vi "PLC_Main_Screen_communication.vi"() -> ()   [LabVIEW 2017]
doc: "Andon System cards scanning and ouput ON/OFF through MQTT protocol. Update data in SQL data base for reporting."
uses:
  Control/Processing_enum.ctl
  Control/Main_Data.ctl
  Control/Andon_demo State.ctl
  <vilib>/addons/database/Connection.llb/Conn ObjectReference.ctl
  <vilib>/NI/Modbus Library/API/master/Modbus Master.lvclass
  Control/Oven_State.ctl
  37ed035b-2b4a-44e1-bf61-a1f42ff74949.vi
  <vilib>/addons/database/Connection.llb/DB Tools Open Connec (Path).vi
  <vilib>/NI/Modbus Library/API/Wrapper/Create TCP Master.vi
  <vilib>/ethernetip/ethernetip.llb/EthernetIP SLC500 Read Bit.vi
  <vilib>/ethernetip/ethernetip.llb/EthernetIP SLC500 Write Bit.vi
  <vilib>/addons/database/NI_Database_API.lvlib
  <vilib>/ethernetip/ethernetip.lvlib
  <vilib>/NI/Modbus Library/API/Wrapper/API Main.lvlib
panel:
  in  "stop":bool
  out "Stop from Main":bool
  out "Change Element":T1(array[cluster])
  out "MACHINE NAME":string[](array[string])
  out "IP Address":string[](array[string])
  in  "Tab Control":enum32{"Oven", "press"}(tab)
  out "Oven Values":u16[][](array[numeric])
  out "Oven live Sql Error":errorcluster
  out "Oven Station ID":string[][](array[string])
  out "Oven LOG SQL Error":errorcluster
  out "LOG Elapsed Time":dbl caption="Elapsed Time (s)"
  out "output cluster":T2
  out "Press Statio ID":string[][](array[string])
  out "Cluster":T3
  out "STATE":T4=enum."PLC_stat"
  out "Shift":i32
  out "CID":string
  out "error out":errorcluster
  out "Deq Element":T5[](array[typedef])
  out "PLC Data":T5[](array[typedef])
  out "Input":bool[](array[boolean])
  # "SERVER for PRESS and OVEN"
  # "1.INPUTS\n2.OUTPUTS\n3.Product code running on system.\n4.Alarms"
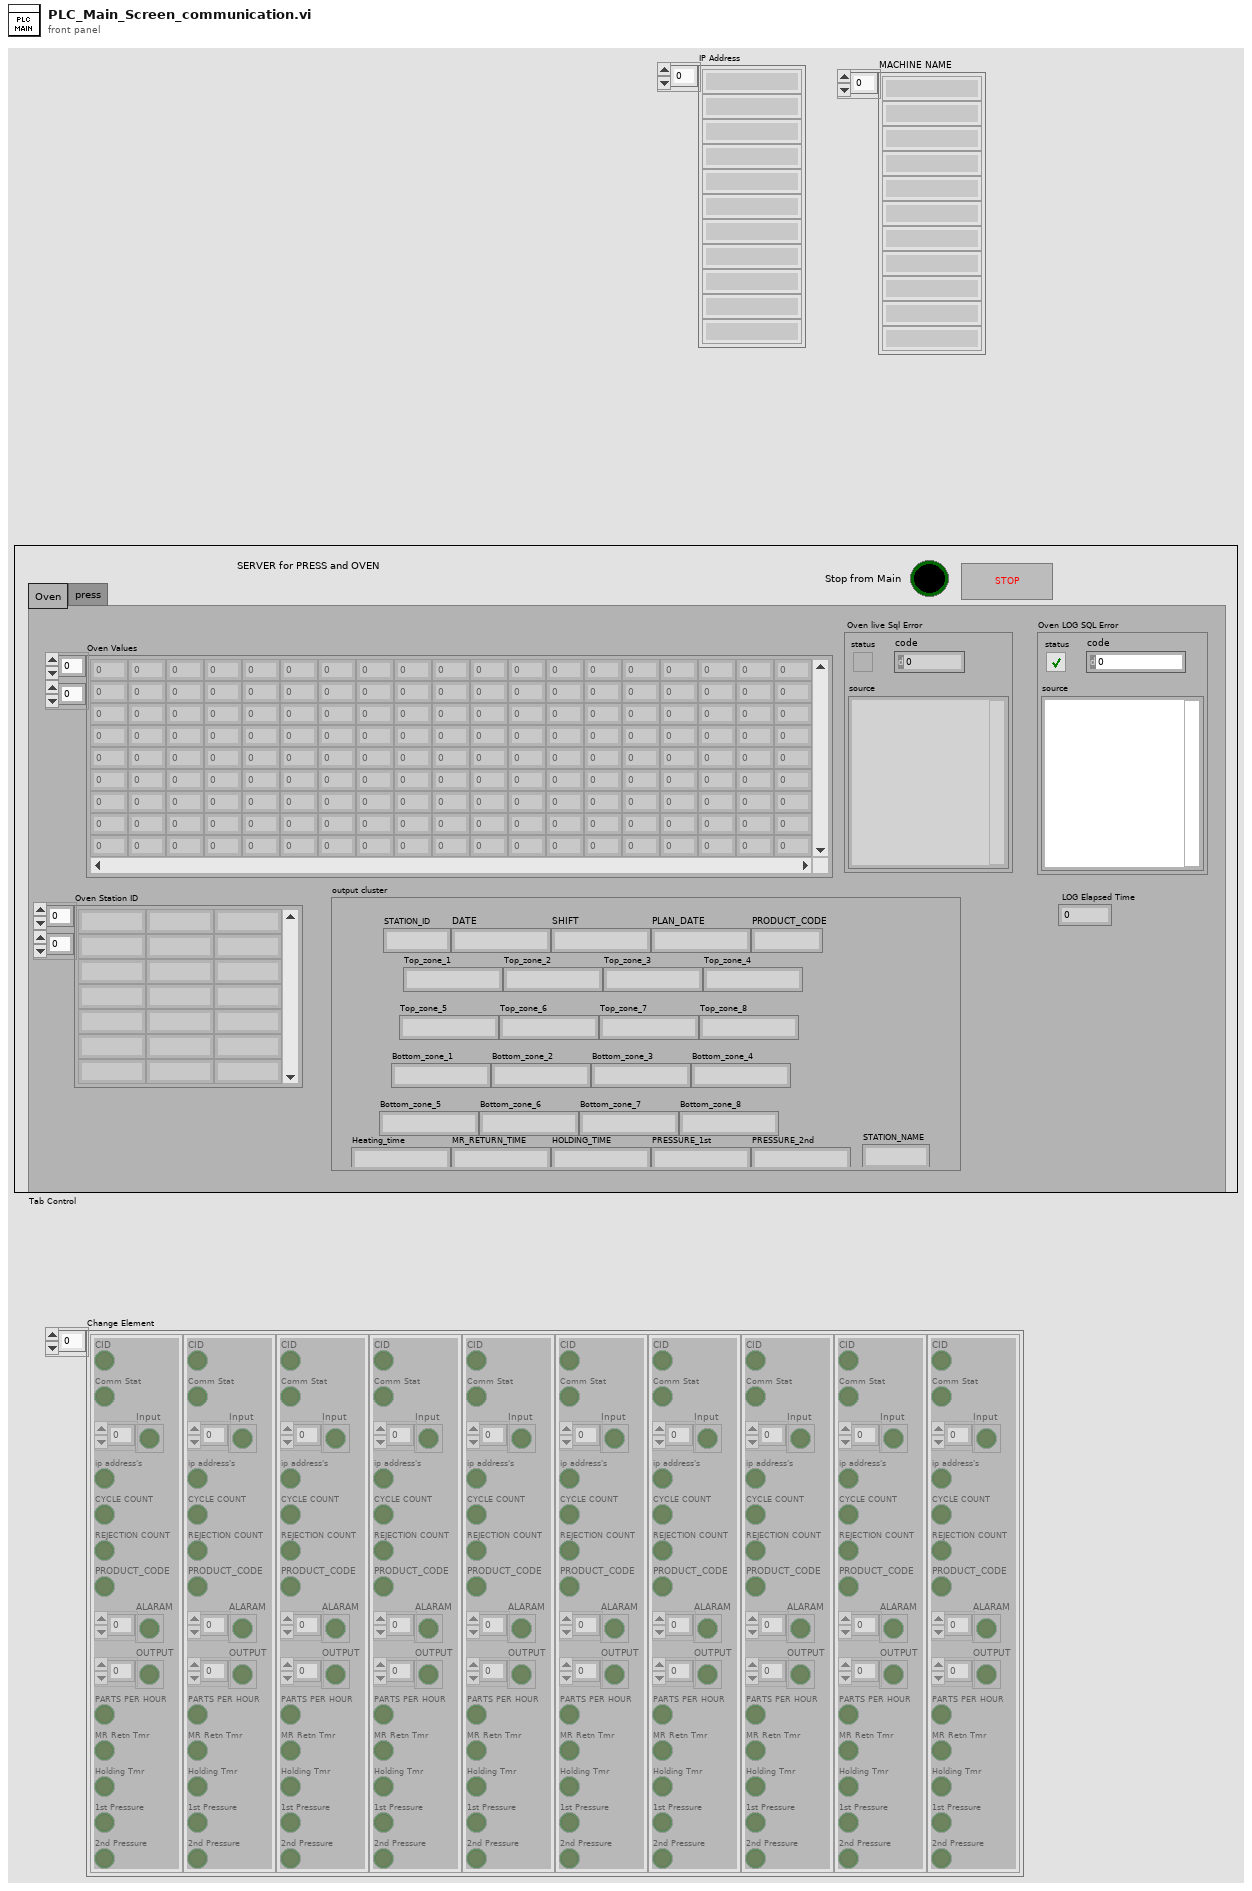
[diagram p1: front panel]
types:
  T1 = cluster{"CID":bool, "Comm Stat":bool, "Input":bool[], "ip address's":bool, "CYCLE COUNT":bool, "REJECTION COUNT":bool, "PRODUCT_CODE":bool, "ALARAM":bool[], "OUTPUT":bool[], "PARTS PER HOUR":bool, "MR Retn Tmr":bool, "Holding Tmr":bool, "1st Pressure":bool, "2nd Pressure":bool}[]
  T2 = cluster{"STATION_ID":string, "DATE":string, "SHIFT":string, "PLAN_DATE":string, "PRODUCT_CODE":string, "Top_zone_1":string, "Top_zone_2":string, "Top_zone_3":string, "Top_zone_4":string, "Top_zone_5":string, "Top_zone_6":string, "Top_zone_7":string, "Top_zone_8":string, "Bottom_zone_1":string, "Bottom_zone_2":string, "Bottom_zone_3":string, "Bottom_zone_4":string, "Bottom_zone_5":string, "Bottom_zone_6":string, "Bottom_zone_7":string, "Bottom_zone_8":string, "Heating_time":string, "MR_RETURN_TIME":string, "HOLDING_TIME":string, "PRESSURE_1st":string, "PRESSURE_2nd":string, "STATION_NAME":string}
  T3 = cluster{"Rejection code":bool[], "Production count":bool[], "Input":bool[][]}
  T4 = typedef "Processing_enum.ctl" = enum16{"Break_down", "Product_Rej_Count", "PLC_stat", "Inita"}
  T5 = typedef "Main_Data.ctl" = cluster{"CID":string, "Comm Stat":bool, "Input":bool[], "ip address's":string, "CYCLE COUNT":u32, "REJECTION COUNT":u32, "PRODUCT_CODE":i16, "ALARAM":bool[], "OUTPUT":bool[], "PARTS PER HOUR":i16, "MR Retn Tmr":dbl, "Holding Tmr":dbl, "1st Pressure":dbl, "2nd Pressure":dbl}
  T6 = enum32{"invalid app kind", "Development System", "Run Time System", "Student Edition", "Embedded LabVIEW", "Evaluation", "Custom"}
  T7 = typedef "Andon_demo State.ctl" = enum16{"Initialise", "Read Inputs", "Process Inputs", "Generate Log Trigger"}
  T8 = typedef "Oven_State.ctl" = enum16{"Initialise", "PLC read", "Live Update", "Log data", "Stop"}
  T9 = typedef "NI_Database_API.lvlib/Conn ObjectReference.ctl" = refnum<k1>
  T10 = cluster{"Oven Number":string[], "Oven NAME":string[], "IP Address":string[], "SQL connection":T9, "Oven Data":u16[][], "PLC ref":refnum<class "Modbus Master.lvclass">[], "Oven Number Txx":string[]}
  T11 = cluster{"CID":string, "Comm Stat":bool, "Input":bool[], "ip address's":string, "CYCLE COUNT":u32, "REJECTION COUNT":u32, "PRODUCT_CODE":i16, "ALARAM":bool[], "OUTPUT":bool[], "PARTS PER HOUR":i16}
  T12 = cluster{"CID":string, "Comm Stat":bool, "Input":bool[], "ip address's":string, "CYCLE COUNT":u32, "REJECTION COUNT":u32, "PRODUCT_CODE":u32, "ALARAM":bool[], "OUTPUT":bool[]}[]
  T13 = typedef "ethernetip.lvlib/ethernetip.ctl" = refnum<k21>
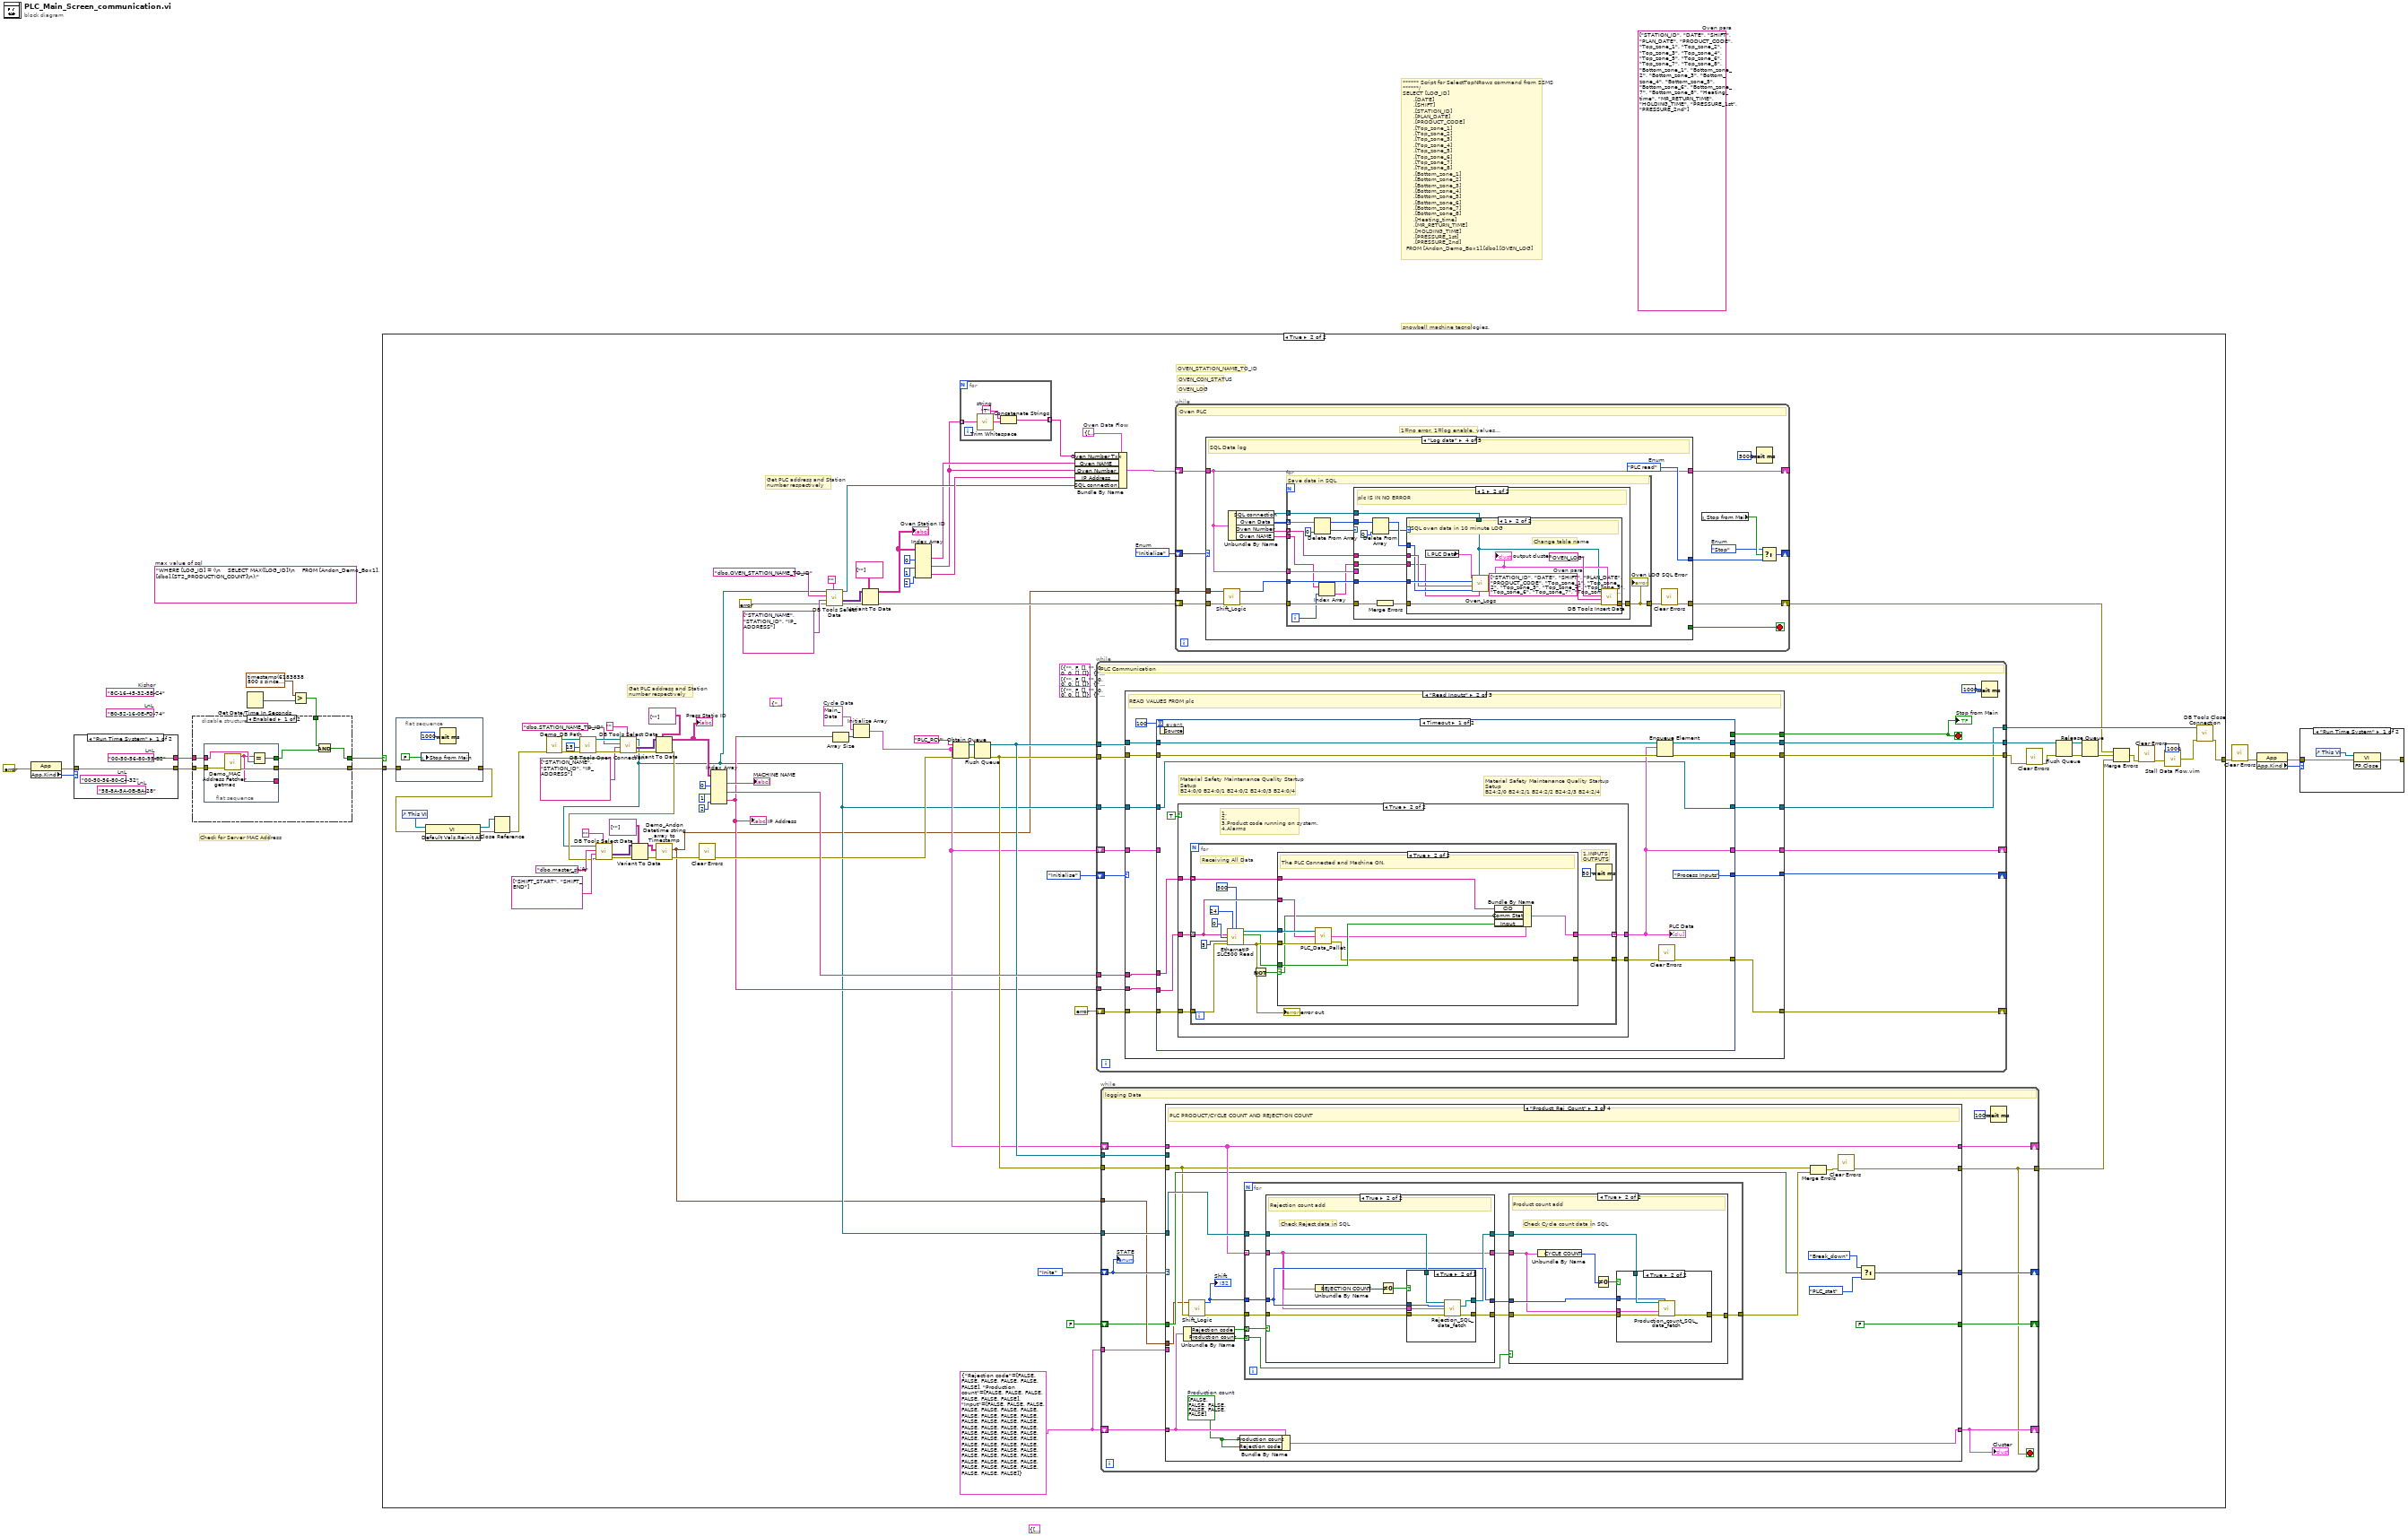
[diagram p0: block diagram]
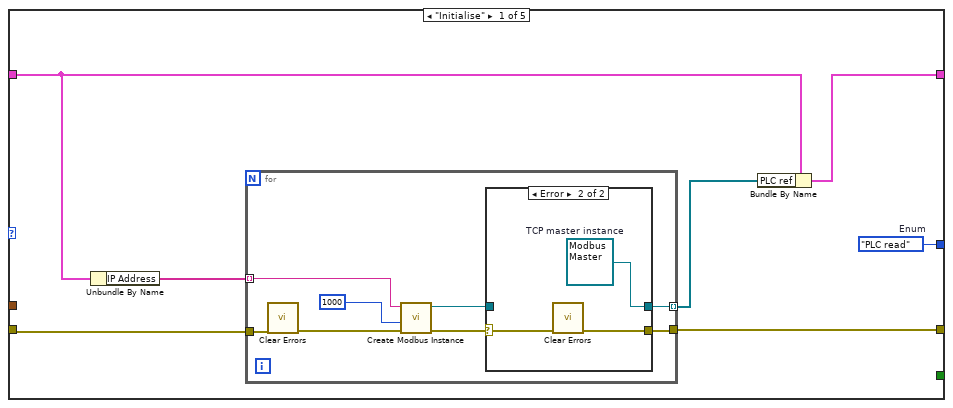
[diagram p3: hidden frame]
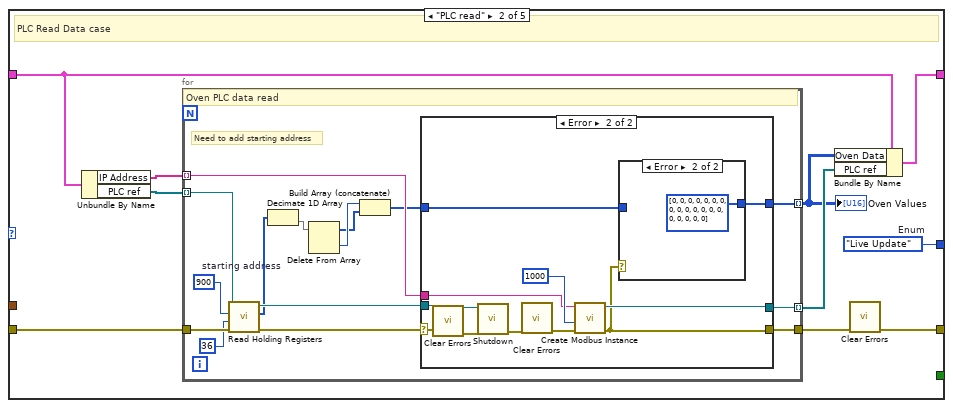
[diagram p5: hidden frame]
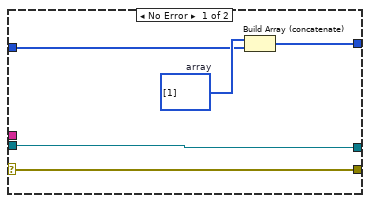
[diagram p6: hidden frame]
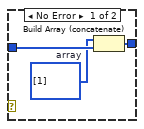
[diagram p7: hidden frame]
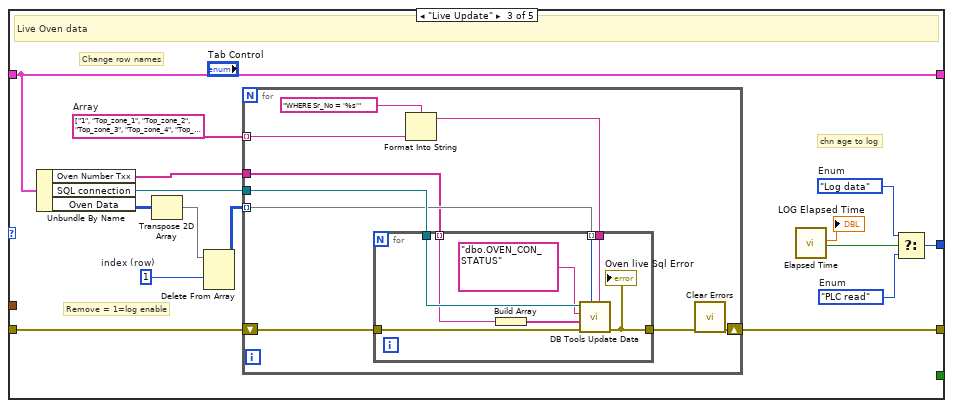
[diagram p8: hidden frame]
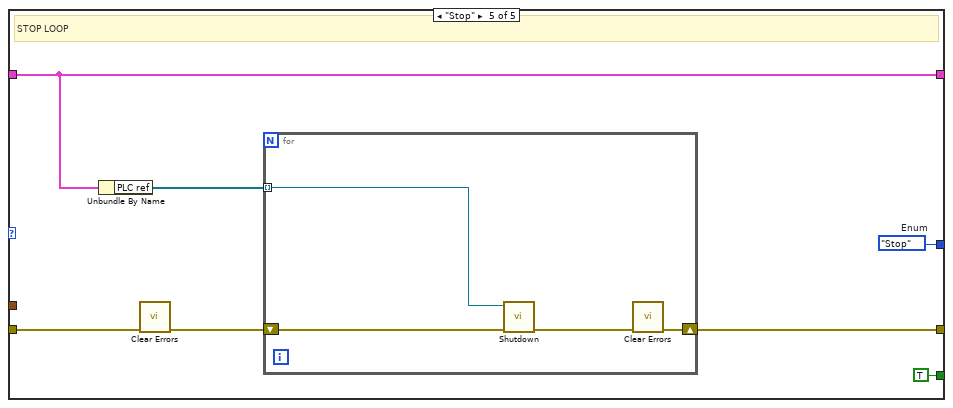
[diagram p11: hidden frame]
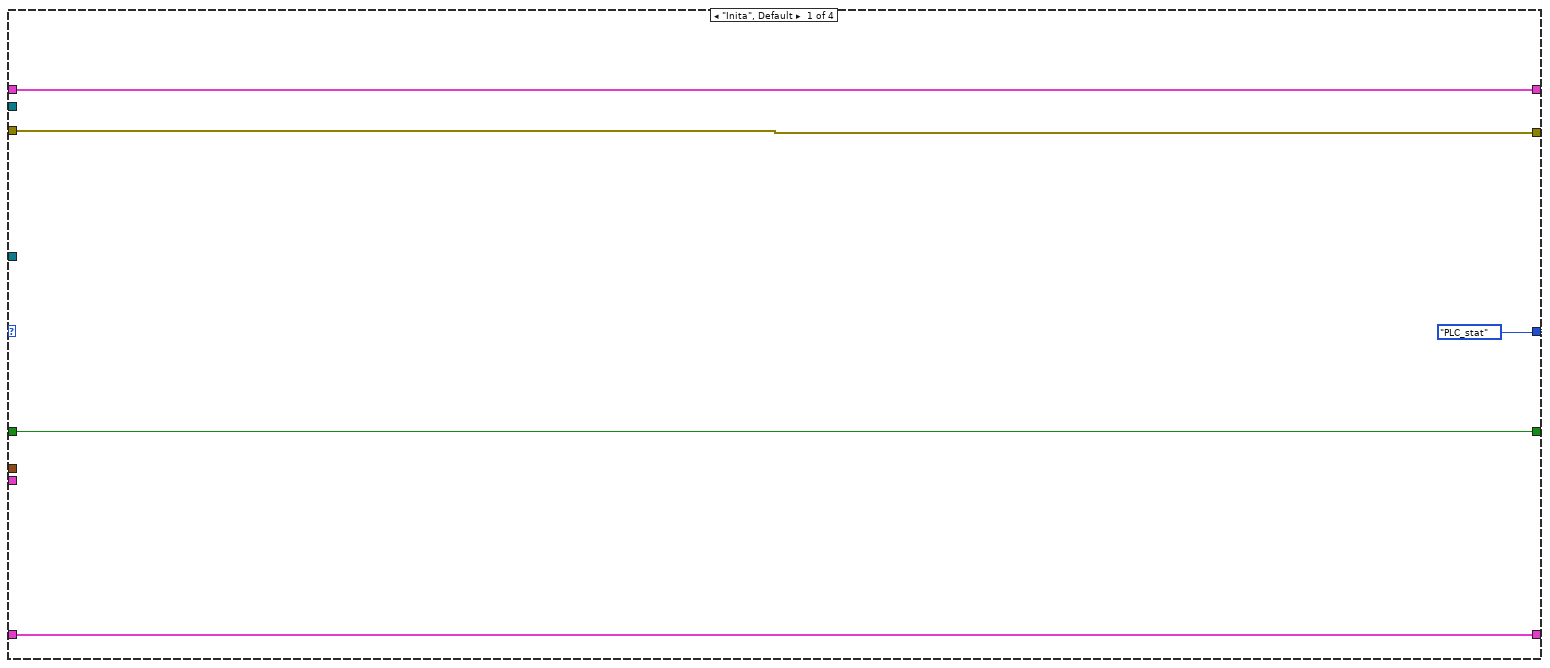
[diagram p12: hidden frame]
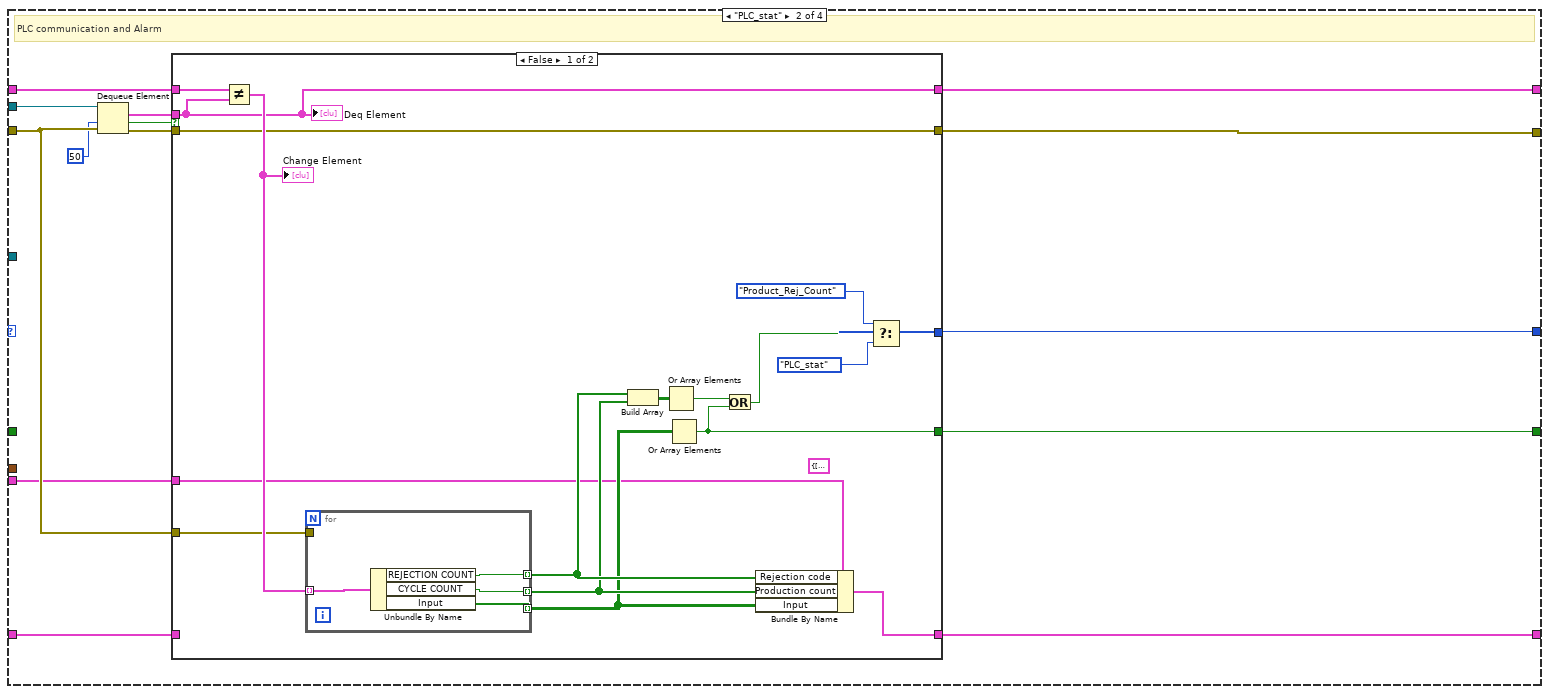
[diagram p13: hidden frame]
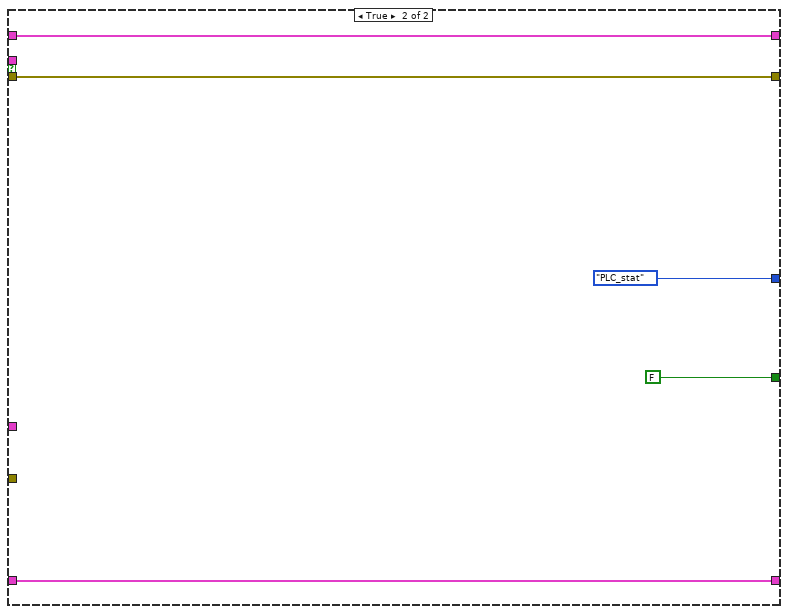
[diagram p14: hidden frame]
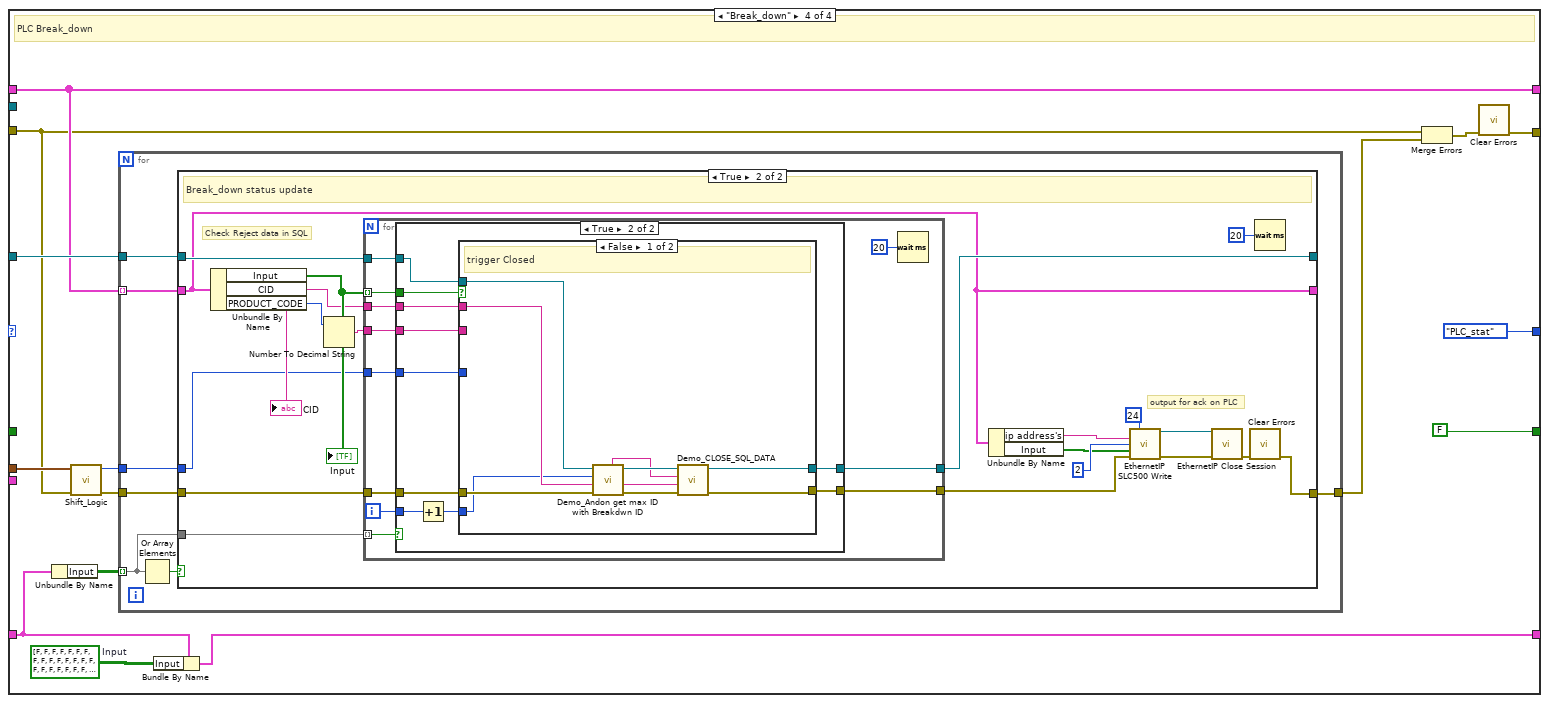
[diagram p19: hidden frame]
diagram:
  (unwired) string[] ["STATION_ID", "DATE", "SHIFT", "PLAN_DATE", "PRODUCT_CODE", "Top_zone_1", "Top_zone_2", "Top_zone_3", "Top_zone_4", "Top_zone_5", "Top_zone_6", "Top_zone_7", "Top_zone_8", "Bottom_zone_1", "Bottom_zone_2", "Bottom_zone_3", "Bottom_zone_4", "Bottom_zone_5", "Bottom_zone_6", "Bottom_zone_7", "Bottom_zone_8", "Heating_time", "MR_RETURN_TIME", "HOLDING_TIME", "PRESSURE_1st", "PRESSURE_2nd"]  # Oven para
  (unwired) "WHERE [LOG_ID] = (\n    SELECT MAX([LOG_ID])\n    FROM [Andon_Demo_Box1].[dbo].[ST2_PRODUCTION_COUNT]\n);"  # max value of sql
  (unwired) T3 {"Rejection code"=[FALSE, FALSE, FALSE, FALSE, FALSE, FALSE, FALSE, FALSE, FALSE, FALSE], "Production count"=[FALSE, FALSE, FALSE, FALSE, FALSE, FALSE, FALSE, FALSE, FALSE, FALSE], "Input"=[[FALSE, FALSE, FALSE, FALSE, FALSE], [FALSE, FALSE, FALSE, FALSE, FALSE], [FALSE, FALSE, FALSE, FALSE, FALSE], [FALSE, FALSE, FALSE, FALSE, FALSE], [FALSE, FALSE, FALSE, FALSE, FALSE], [FALSE, FALSE, FALSE, FALSE, FALSE], [FALSE, FALSE, FALSE, FALSE, FALSE], [FALSE, FALSE, FALSE, FALSE, FALSE], [FALSE, FALSE, FALSE, FALSE, FALSE], [FALSE, FALSE, FALSE, FALSE, FALSE]]}
  (unwired) "B0-52-16-0E-FD-74"  # LnL
  (unwired) "8C-16-45-32-5B-C4"  # Kishor
  # "****** Script for SelectTopNRows command from SSMS  ******/\nSELECT [LOG_ID]\n      ,[DATE]\n      ,[SHIFT]\n      ,[STATION_ID]\n      ,[PLAN_DATE]\n      ,[PRODUCT_CODE]\n      ,[Top_zone_1]\n      ,[Top_zone_2]\n      ,[Top_zone_3]\n      ,[Top_zone_4]\n      ,[Top_zone_5]\n      ,[Top_zone_6]\n      ,[Top_zone_7]\n      ,[Top_zone_8]\n      ,[Bottom_zone_1]\n      ,[Bottom_zone_2]\n      ,[Bottom_zone_3]\n      ,[Bottom_zone_4]\n      ,[Bottom_zone_5]\n      ,[Bottom_zone_6]\n      ,[Bottom_zone_7]\n      ,[Bottom_zone_8]\n      ,[Heating_time]\n      ,[MR_RETURN_TIME]\n      ,[HOLDING_TIME]\n      ,[PRESSURE_1st]\n      ,[PRESSURE_2nd]\n  FROM [Andon_Demo_Box1].[dbo].[OVEN_LOG]"
  # "snowbell machine tecnologies."
  # "Check for Server MAC Address"
  n1 = property class="App"(error in=errorcluster {"status"=FALSE, "code"=0, "source"=""} ("error in (no error)")) -> (error out=w10:errorcluster, "App.Kind"=w9:T6)  [unwired: 1 in, 1 out]
  n2 = case shown="\"Run Time System\"" w9 {
    tunnel: [w16 w18] -> w7
    tunnel: w10 -> [w16 w18]
    tunnel: [w15 w17] -> w6
    frame "Run Time System" {
      (unwired) "00-50-56-80-C4-32"  # LnL
      w15 = "00-50-56-80-95-B2"  # LnL
      (unwired) "58-8A-5A-0B-BA-28"  # LnL
    }
    frame "Development System", Default {
      w17 = "28-D2-44-6F-84-04"  # ASIM LAPTOP
    }
  }
  n3 = Get Date/Time In Seconds() -> (seconds since 1Jan1904=w1:timestamp)
  n4 = Greater?(x=timestamp(6183838800 s since 1904-01-01), y=w1) -> (0:w3:bool)
  n5 = disable-structure shown="Enabled" {
    disable-tunnel: [w21 TRUE] -> w12
    disable-tunnel: [w24 w30] -> w11
    disable-tunnel: w7 -> [w23 w30]
    disable-tunnel: w6 -> [w22 _]
    disable-tunnel: w3 -> [w19 _]
    frame Enabled {
      n6 = flat-sequence {
        tunnel: w23 -> [w29]
        tunnel: [w27] -> w20
        tunnel: [w28] -> w24
        tunnel: w22 -> [w26]
        tunnel: [w25] -> _
        frame #0 {
          n7 = call "Demo_MAC Address Fetcher getmac.vi"("error in (no error)"=w29) -> ("error out"=w28:errorcluster, "First Matched MAC"=w25:string)  [unwired: 6 in, 3 out]
          n8 = Equal?(x=w25, y=w26) -> (x = y?=w27:bool)
        }
      }
      n9 = And(x=w19, y=w20) -> (x .and. y?=w21:bool)
    }
    frame Disabled {
    }
  }
  n10 = case shown="True" w12 {
    tunnel: w11 -> [w32 w102]
    tunnel: [w32 w65] -> w4
    frame False {
    }
    frame True {
      w38 = Oven_State."Initialise"  # Enum
      w54 = T10 {"Oven Number"=[], "Oven NAME"=[], "IP Address"=[], "SQL connection"=refnum, "Oven Data"=[], "PLC ref"=[], "Oven Number Txx"=[]}  # Oven Data Flow
      w57 = T5 {"CID"="", "Comm Stat"=FALSE, "Input"=[FALSE, FALSE, FALSE, FALSE, FALSE], "ip address's"="", "CYCLE COUNT"=0, "REJECTION COUNT"=0, "PRODUCT_CODE"=0, "ALARAM"=[FALSE, FALSE, FALSE, FALSE, FALSE, FALSE, FALSE, FALSE], "OUTPUT"=[FALSE, FALSE, FALSE, FALSE, FALSE], "PARTS PER HOUR"=0, "MR Retn Tmr"=0.0, "Holding Tmr"=0.0, "1st Pressure"=0.0, "2nd Pressure"=0.0}  # Cycle Data
      (unwired) T11 {"CID"="", "Comm Stat"=FALSE, "Input"=[FALSE, FALSE, FALSE, FALSE, FALSE], "ip address's"="", "CYCLE COUNT"=0, "REJECTION COUNT"=0, "PRODUCT_CODE"=0, "ALARAM"=[FALSE, FALSE, FALSE, FALSE, FALSE, FALSE, FALSE, FALSE], "OUTPUT"=[FALSE, FALSE, FALSE, FALSE, FALSE], "PARTS PER HOUR"=0} ("constatnt")
      w56 = T3 {"Rejection code"=[FALSE, FALSE, FALSE, FALSE, FALSE, FALSE], "Production count"=[FALSE, FALSE, FALSE, FALSE, FALSE, FALSE], "Input"=[[FALSE, FALSE, FALSE, FALSE, FALSE], [FALSE, FALSE, FALSE, FALSE, FALSE], [FALSE, FALSE, FALSE, FALSE, FALSE], [FALSE, FALSE, FALSE, FALSE, FALSE], [FALSE, FALSE, FALSE, FALSE, FALSE], [FALSE, FALSE, FALSE, FALSE, FALSE], [FALSE, FALSE, FALSE, FALSE, FALSE], [FALSE, FALSE, FALSE, FALSE, FALSE], [FALSE, FALSE, FALSE, FALSE, FALSE], [FALSE, FALSE, FALSE, FALSE, FALSE]]}
      (unwired) T12 [{"CID"="", "Comm Stat"=FALSE, "Input"=[], "ip address's"="", "CYCLE COUNT"=0, "REJECTION COUNT"=0, "PRODUCT_CODE"=0, "ALARAM"=[], "OUTPUT"=[]}, {"CID"="", "Comm Stat"=FALSE, "Input"=[], "ip address's"="", "CYCLE COUNT"=0, "REJECTION COUNT"=0, "PRODUCT_CODE"=0, "ALARAM"=[], "OUTPUT"=[]}, {"CID"="", "Comm Stat"=FALSE, "Input"=[], "ip address's"="", "CYCLE COUNT"=0, "REJECTION COUNT"=0, "PRODUCT_CODE"=0, "ALARAM"=[], "OUTPUT"=[]}, {"CID"="", "Comm Stat"=FALSE, "Input"=[], "ip address's"="", "CYCLE COUNT"=0, "REJECTION COUNT"=0, "PRODUCT_CODE"=0, "ALARAM"=[], "OUTPUT"=[]}, {"CID"="", "Comm Stat"=FALSE, "Input"=[], "ip address's"="", "CYCLE COUNT"=0, "REJECTION COUNT"=0, "PRODUCT_CODE"=0, "ALARAM"=[], "OUTPUT"=[]}, {"CID"="", "Comm Stat"=FALSE, "Input"=[], "ip address's"="", "CYCLE COUNT"=0, "REJECTION COUNT"=0, "PRODUCT_CODE"=0, "ALARAM"=[], "OUTPUT"=[]}, {"CID"="", "Comm Stat"=FALSE, "Input"=[], "ip address's"="", "CYCLE COUNT"=0, "REJECTION COUNT"=0, "PRODUCT_CODE"=0, "ALARAM"=[], "OUTPUT"=[]}, {"CID"="", "Comm Stat"=FALSE, "Input"=[], "ip address's"="", "CYCLE COUNT"=0, "REJECTION COUNT"=0, "PRODUCT_CODE"=0, "ALARAM"=[], "OUTPUT"=[]}, {"CID"="", "Comm Stat"=FALSE, "Input"=[], "ip address's"="", "CYCLE COUNT"=0, "REJECTION COUNT"=0, "PRODUCT_CODE"=0, "ALARAM"=[], "OUTPUT"=[]}, {"CID"="", "Comm Stat"=FALSE, "Input"=[FALSE, FALSE, FALSE, FALSE, FALSE], "ip address's"="", "CYCLE COUNT"=0, "REJECTION COUNT"=0, "PRODUCT_CODE"=0, "ALARAM"=[FALSE, FALSE, FALSE, FALSE, FALSE, FALSE, FALSE, FALSE], "OUTPUT"=[FALSE, FALSE, FALSE, FALSE, FALSE]}]
      (unwired) T12 [{"CID"="", "Comm Stat"=FALSE, "Input"=[], "ip address's"="", "CYCLE COUNT"=0, "REJECTION COUNT"=0, "PRODUCT_CODE"=0, "ALARAM"=[], "OUTPUT"=[]}, {"CID"="", "Comm Stat"=FALSE, "Input"=[], "ip address's"="", "CYCLE COUNT"=0, "REJECTION COUNT"=0, "PRODUCT_CODE"=0, "ALARAM"=[], "OUTPUT"=[]}, {"CID"="", "Comm Stat"=FALSE, "Input"=[], "ip address's"="", "CYCLE COUNT"=0, "REJECTION COUNT"=0, "PRODUCT_CODE"=0, "ALARAM"=[], "OUTPUT"=[]}, {"CID"="", "Comm Stat"=FALSE, "Input"=[], "ip address's"="", "CYCLE COUNT"=0, "REJECTION COUNT"=0, "PRODUCT_CODE"=0, "ALARAM"=[], "OUTPUT"=[]}, {"CID"="", "Comm Stat"=FALSE, "Input"=[], "ip address's"="", "CYCLE COUNT"=0, "REJECTION COUNT"=0, "PRODUCT_CODE"=0, "ALARAM"=[], "OUTPUT"=[]}, {"CID"="", "Comm Stat"=FALSE, "Input"=[], "ip address's"="", "CYCLE COUNT"=0, "REJECTION COUNT"=0, "PRODUCT_CODE"=0, "ALARAM"=[], "OUTPUT"=[]}, {"CID"="", "Comm Stat"=FALSE, "Input"=[], "ip address's"="", "CYCLE COUNT"=0, "REJECTION COUNT"=0, "PRODUCT_CODE"=0, "ALARAM"=[], "OUTPUT"=[]}, {"CID"="", "Comm Stat"=FALSE, "Input"=[], "ip address's"="", "CYCLE COUNT"=0, "REJECTION COUNT"=0, "PRODUCT_CODE"=0, "ALARAM"=[], "OUTPUT"=[]}, {"CID"="", "Comm Stat"=FALSE, "Input"=[], "ip address's"="", "CYCLE COUNT"=0, "REJECTION COUNT"=0, "PRODUCT_CODE"=0, "ALARAM"=[], "OUTPUT"=[]}, {"CID"="", "Comm Stat"=FALSE, "Input"=[FALSE, FALSE, FALSE, FALSE, FALSE], "ip address's"="", "CYCLE COUNT"=0, "REJECTION COUNT"=0, "PRODUCT_CODE"=0, "ALARAM"=[FALSE, FALSE, FALSE, FALSE, FALSE, FALSE, FALSE, FALSE], "OUTPUT"=[FALSE, FALSE, FALSE, FALSE, FALSE]}]
      (unwired) T12 [{"CID"="", "Comm Stat"=FALSE, "Input"=[], "ip address's"="", "CYCLE COUNT"=0, "REJECTION COUNT"=0, "PRODUCT_CODE"=0, "ALARAM"=[], "OUTPUT"=[]}, {"CID"="", "Comm Stat"=FALSE, "Input"=[], "ip address's"="", "CYCLE COUNT"=0, "REJECTION COUNT"=0, "PRODUCT_CODE"=0, "ALARAM"=[], "OUTPUT"=[]}, {"CID"="", "Comm Stat"=FALSE, "Input"=[], "ip address's"="", "CYCLE COUNT"=0, "REJECTION COUNT"=0, "PRODUCT_CODE"=0, "ALARAM"=[], "OUTPUT"=[]}, {"CID"="", "Comm Stat"=FALSE, "Input"=[], "ip address's"="", "CYCLE COUNT"=0, "REJECTION COUNT"=0, "PRODUCT_CODE"=0, "ALARAM"=[], "OUTPUT"=[]}, {"CID"="", "Comm Stat"=FALSE, "Input"=[], "ip address's"="", "CYCLE COUNT"=0, "REJECTION COUNT"=0, "PRODUCT_CODE"=0, "ALARAM"=[], "OUTPUT"=[]}, {"CID"="", "Comm Stat"=FALSE, "Input"=[], "ip address's"="", "CYCLE COUNT"=0, "REJECTION COUNT"=0, "PRODUCT_CODE"=0, "ALARAM"=[], "OUTPUT"=[]}, {"CID"="", "Comm Stat"=FALSE, "Input"=[], "ip address's"="", "CYCLE COUNT"=0, "REJECTION COUNT"=0, "PRODUCT_CODE"=0, "ALARAM"=[], "OUTPUT"=[]}, {"CID"="", "Comm Stat"=FALSE, "Input"=[], "ip address's"="", "CYCLE COUNT"=0, "REJECTION COUNT"=0, "PRODUCT_CODE"=0, "ALARAM"=[], "OUTPUT"=[]}, {"CID"="", "Comm Stat"=FALSE, "Input"=[], "ip address's"="", "CYCLE COUNT"=0, "REJECTION COUNT"=0, "PRODUCT_CODE"=0, "ALARAM"=[], "OUTPUT"=[]}, {"CID"="", "Comm Stat"=FALSE, "Input"=[FALSE, FALSE, FALSE, FALSE, FALSE], "ip address's"="", "CYCLE COUNT"=0, "REJECTION COUNT"=0, "PRODUCT_CODE"=0, "ALARAM"=[FALSE, FALSE, FALSE, FALSE, FALSE], "OUTPUT"=[FALSE, FALSE, FALSE, FALSE, FALSE]}]
      # "OVEN_LOG"
      # "OVEN_CON_STATUS"
      # "OVEN_STATION_NAME_TO_ID"
      # "Get PLC address and Station\nnumber respectively"
      # "Get PLC address and Station\nnumber respectively"
      n11 = flat-sequence {
        tunnel: [w504] -> w106
        tunnel: w102 -> [w504]
        frame #0 {
          n12 = local write "Stop from Main"(FALSE ("stop")) -> ()
          n13 = Wait (ms)(milliseconds to wait=u32 1000) -> ()  [unwired: 1 out]
        }
      }
      n14 = control-ref of="This VI"() -> (w105:refnum<vi>)
      n15 = invoke class="VI" method="Default Vals.Reinit All"(reference=w105, error in=w106) -> (reference out=w104:refnum<vi>, error out=w103:errorcluster)  [unwired: 1 in, 1 out]
      n16 = Close Reference(reference=w104, error in (no error)=w103) -> (error out=w107:errorcluster)
      n17 = call "Demo_DB Path.vi"("error in"=w107) -> ("error out"=w95:errorcluster, "DB Path"=w96:path)  [unwired: 9 in]
      n18 = call-poly <vilib>:"DB Tools Open Connection.vi"("error in (no error)"=w95, "connection timeout (15)"=15, "connection information"=w96) -> ("error out"=w100:errorcluster, "connection reference"=w99:T9)  [unwired: 5 in]
      n19 = call <vilib>:"DB Tools Select Data.vi"("condition"="", "error in (no error)"=w100, "columns"=string[] ["STATION_NAME", "STATION_ID", "IP_ADDRESS"], "table"="dbo.STATION_NAME_TO_ID", "connection reference"=w99) -> ("error out"=w97:errorcluster, "data"=w98:variant[][], "connection reference out"=w43:T9)  [unwired: 1 in]
      n20 = Variant To Data(error in=w97, type=string[][] [[""]], Variant=w98) -> (data=w89:string[][], error out=w73:errorcluster)
      "Press Statio ID" <- w89
      n21 = call <vilib>:"DB Tools Select Data.vi"("condition"="", "error in (no error)"=w73, "columns"=string[] ["SHIFT_START", "SHIFT_END"], "table"="dbo.master_shift", "connection reference"=w43) -> ("error out"=w79:errorcluster, "data"=w77:variant[][])  [unwired: 1 in, 1 out]
      n22 = Variant To Data(error in=w79, type=string[][] [[""]], Variant=w77) -> (data=w76:string[][], error out=w75:errorcluster)
      n23 = call "Demo_Andon Datetime string array to Timestamp.vi"("error in (no error)"=w75, "String Array In"=w76) -> ("error out"=w74:errorcluster, "Time Stamp Out"=w33:timestamp[])  [unwired: 8 in]
      n24 = call <vilib>:"Clear Errors.vi"("error in (no error)"=w74) -> ("error out"=w72:errorcluster)  [unwired: 5 in, 1 out]
      n25 = Index Array(array=w89, index (col) #1=0 ("disabled index (col)"), index (col) #2=1 ("disabled index (col)"), index (col) #3=2 ("disabled index (col)")) -> (element #1=→"MACHINE NAME":string[], element #2=w85:string[], element #3=w63:string[])  [unwired: 3 in]
      "IP Address" <- w63
      n26 = call <vilib>:"DB Tools Select Data.vi"("condition"="", "error in (no error)"=errorcluster {"status"=FALSE, "code"=0, "source"=""}, "columns"=string[] ["STATION_NAME", "STATION_ID", "IP_ADDRESS"], "table"="dbo.OVEN_STATION_NAME_TO_ID", "connection reference"=w43) -> ("error out"=w45:errorcluster, "data"=w44:variant[][], "connection reference out"=w39:T9)  [unwired: 1 in]
      n27 = Array Size(array=w63) -> (size(s)=w62:i32)
      n28 = Initialize Array(w57, w62) -> (w61:T5[])
      n29 = Variant To Data(error in=w45, type=string[][] [[""]], Variant=w44) -> (data=w50:string[][], error out=w41:errorcluster)
      "Oven Station ID" <- w50
      n30 = Index Array(array=w50, index (col) #1=0 ("disabled index (col)"), index (col) #2=1 ("disabled index (col)"), index (col) #3=2 ("disabled index (col)")) -> (element #1=w37:string[], element #2=w35:string[], element #3=w40:string[])  [unwired: 3 in]
      n31 = Obtain Queue(name (unnamed)="PLC_RCV", element data type=w61, error in (no error)=w72) -> (queue out=w112:refnum<queue>, error out=w111:errorcluster)  [unwired: 2 in, 1 out]
      n32 = for {
        tunnel: w35 -> [w118] mode=indexing
        tunnel: [w117] -> w36 mode=indexing
        w119 = "T"  # string
        n33 = call <vilib>:"Trim Whitespace.vi"("string"=w118) -> ("trimmed string"=w120:string)  [unwired: 1 in]
        n34 = Concatenate Strings(w119, w120) -> (w117:string)
      }
      n35 = Flush Queue(queue=w112, error in (no error)=w111) -> (queue out=w68:refnum<queue>, error out=w67:errorcluster)  [unwired: 1 out]
      n36 = Bundle By Name(cluster=w54, "Oven Number Txx"=w36, "Oven NAME"=w37, "Oven Number"=w35, "IP Address"=w40, "SQL connection"=w39) -> (w55:T10)
      n37 = while {
        tunnel: w67 -> [w521]
        tunnel: [w520] -> w110
        tunnel: w68 -> [w519]
        tunnel: [w518] -> w113
        shift-right: [w515] -> _
        shift-left: errorcluster {"status"=FALSE, "code"=0, "source"=""} ("error in (no error) 2") -> [w516]
        tunnel: w63 -> [w514]
        tunnel: w85 -> [w513]
        shift-right: [w511] -> _
        shift-left: w61 -> [w510]
        tunnel: w43 -> [w509]
        tunnel: [w508] -> w64
        shift-right: [w507] -> _
        shift-left: Andon_demo_State."Initialise" -> [w512]
        stop <- w517 stop-if-true
        # "PLC Communication"
        n38 = case shown="\"Read Inputs\"" w512 {
          tunnel: w521 -> [w526 w542 w615]
          tunnel: [w526 w541 w615] -> w520
          tunnel: w519 -> [w527 w540 w614]
          tunnel: [w527 w539 w614] -> w518
          tunnel: [_ w538 _] -> w517
          tunnel: w516 -> [w524 w537 w613]
          tunnel: [w524 w536 w612] -> w515
          tunnel: w514 -> [_ w535 _]
          tunnel: w513 -> [_ w534 _]
          tunnel: [w525 w532 w611] -> w511
          tunnel: w510 -> [w525 w528 w609]
          tunnel: w509 -> [w523 w530 w608]
          tunnel: [w523 w529 w608] -> w508
          tunnel: [Andon_demo_State."Read Inputs" w531 Andon_demo_State."Read Inputs"] -> w507
          frame "Initialise", Default {
          }
          frame "Read Inputs" {
            # "READ VALUES FROM plc"
            n39 = event shown="[0] Timeout" {
              selector: _ -> [_ _]
              dyn-events: _ -> [_ _]
              timeout: 100 -> [_ _]
              tunnel: [_ w604] -> w538
              tunnel: [w552 w606] -> w541
              tunnel: w542 -> [w553 w606]
              tunnel: [w554 w605] -> w539
              tunnel: w540 -> [w555 w605]
              tunnel: w537 -> [w550 _]
              tunnel: [w548 w603] -> w536
              tunnel: w535 -> [w551 _]
              tunnel: w534 -> [w549 _]
              tunnel: [w546 _] -> w532
              tunnel: [Andon_demo_State."Process Inputs" Andon_demo_State."Initialise"] -> w531
              tunnel: [w544 w600] -> w529
              tunnel: w530 -> [w544 w600]
              tunnel: w528 -> [_ _]
              event Timeout {
                # "Material\tSafety\tMaintenance\tQuality\tStartup Setup\nB24:2/0\tB24:2/1\tB24:2/2\tB24:2/3\tB24:2/4"
                # "Material\tSafety\tMaintenance\tQuality\tStartup Setup\nB24:0/0\tB24:0/1\tB24:0/2\tB24:0/3\tB24:0/4"
                n40 = event-data() -> ()  [unwired: 1 in, 1 out]
                n41 = case shown="True" TRUE {
                  tunnel: w551 -> [_ w563]
                  tunnel: w550 -> [w557 w562]
                  tunnel: w549 -> [_ w561]
                  tunnel: [w558 w560] -> w547
                  tunnel: [w556 w559] -> w546
                  frame False {
                    n42 = call "TESTING DUMMY PLC.vi"("error in (no error)"=w557) -> ("error out"=w558:errorcluster, "PLC Simu OUT"=w556:T5[])  [unwired: 9 in]
                  }
                  frame True {
                    # "1.\n2.\n3.Product code running on system.\n4.Alarms"
                    n43 = for {
                      tunnel: w563 -> [w572] mode=indexing
                      tunnel: w562 -> [w576]
                      tunnel: [w565] -> w559 mode=indexing
                      tunnel: w561 -> [w564] mode=indexing
                      tunnel: [w573] -> w560
                      # "1.INPUTS OUTPUTS"
                      # "Receiving All Data"
                      n44 = call-poly <vilib>:"EthernetIP SLC500 Read.vi"("File Number"=u16 24, "Timeout (ms)"=500, "Network Path"=w572, "Element Number"=u16 0, "Number of Bits"=u32 5 ("Number of Bytes"), "error in"=w576) -> ("Session out"=w567:T13, "Data"=w566:bool[], "error out"=w571:errorcluster)  [unwired: 7 in]
                      "error out" <- w571
                      n45 = Not(x=w571) -> (.not. x?=w570:bool)
                      n46 = case shown="True" w570 {
                        selector: w570 -> [w584 w595]
                        tunnel: [w590 w591] -> w573
                        tunnel: w572 -> [w586 w597]
                        tunnel: w571 -> [w588 w599]
                        tunnel: w567 -> [w589 w598]
                        tunnel: w566 -> [_ w596]
                        tunnel: [w580 w594] -> w565
                        tunnel: w564 -> [w585 w593]
                        frame False {
                          w579 = T5 {"CID"="", "Comm Stat"=FALSE, "Input"=[FALSE, FALSE, FALSE, FALSE, FALSE], "ip address's"="", "CYCLE COUNT"=0, "REJECTION COUNT"=0, "PRODUCT_CODE"=0, "ALARAM"=[FALSE, FALSE, FALSE, FALSE, FALSE, FALSE, FALSE, FALSE], "OUTPUT"=[FALSE, FALSE, FALSE, FALSE, FALSE], "PARTS PER HOUR"=0, "MR Retn Tmr"=0.0, "Holding Tmr"=0.0, "1st Pressure"=0.0, "2nd Pressure"=0.0}  # Cycle Data
                          w578 = u16 0
                          # "The PLC is not connected or machine OFF"
                          n47 = call <vilib>:"Clear Errors.vi"("error in (no error)"=w588) -> ("error out"=w587:errorcluster)  [unwired: 5 in, 1 out]
                          n48 = call <vilib>:"EthernetIP Close Session.vi"("error in"=w587, "Session in"=w589) -> ("error out"=w590:errorcluster)  [unwired: 9 in]
                          n49 = Bundle By Name(cluster=w579, "PARTS PER HOUR"=w578, "ip address's"=w586, "CID"=w585, "Comm Stat"=w584, "Input"=bool[] [FALSE, FALSE, FALSE, FALSE, FALSE] ("Data"), "CYCLE COUNT"=w578, "REJECTION COUNT"=w578, "PRODUCT_CODE"=w578, "ALARAM"=bool[] [FALSE, FALSE, FALSE, FALSE, FALSE, FALSE, FALSE, FALSE] ("Data"), "OUTPUT"=bool[] [FALSE, FALSE, FALSE, FALSE, FALSE] ("Data")) -> (w580:T5)
                        }
                        frame True {
                          # "The PLC Connected and Machine ON."
                          n50 = call "PLC_Data_Pallet.vi"("error in (no error)"=w599, "condition"=w597, "Refnum in"=w598) -> ("error out"=w591:errorcluster, "output cluster"=w592:T5)  [unwired: 1 in]
                          n51 = Bundle By Name(cluster=w592, "CID"=w593, "Comm Stat"=w595, "Input"=w596) -> (w594:T5)
                        }
                      }
                      n52 = Wait (ms)(milliseconds to wait=u32 50) -> ()  [unwired: 1 out]
                    }
                  }
                }
                "PLC Data" <- w546
                n53 = Enqueue Element(queue=w555, element=w546, error in (no error)=w553) -> (queue out=w554:refnum<queue>, error out=w552:errorcluster)  [unwired: 1 in, 1 out]
                n54 = call <vilib>:"Clear Errors.vi"("error in (no error)"=w547) -> ("error out"=w548:errorcluster)  [unwired: 5 in, 1 out]
              }
              event "stop": Value Change {
                n55 = event-data() -> ()  [unwired: 1 in, 1 out]
                n56 = call "Login to stop exe.vi"("error in (no error) 2"=errorcluster {"status"=FALSE, "code"=0, "source"=""}) -> ("error in (no error)"=w603:errorcluster, "Success"=w604:bool)  [unwired: 7 in]
              }
            }
          }
          frame "Process Inputs" {
            # "put data in SQl if PLC station is in error"
            n57 = for {
              tunnel: w613 -> [w631]
              tunnel: [w629] -> w611
              tunnel: w609 -> [w616] mode=indexing
              tunnel: w608 -> [w632]
              tunnel: [w630] -> w610
              tunnel: w609 -> [w629]
              w617 = "CON_STATUS" ("table")
              # "PLC com Nok"
              # "PLC com ok"
              # "output for ack on PLC"
              n58 = Unbundle By Name(w616) -> ("Comm Stat"=w633:bool)
              n59 = Unbundle By Name(w616) -> ("CID"=w627:string, "ALARAM"=w621:bool[])
              n60 = Concatenate Strings("T" ("string"), w627) -> (w626:string)
              n61 = Build Array(w626) -> (w622:string[])
              n62 = Select(t=1, s=w633, f=0 ("t")) -> (s? t:f=w618:i32)
              n63 = call <vilib>:"DB Tools Update Data.vi"("condition"="WHERE Sr_No = 1", "data"=w618, "error in (no error)"=w631, "columns"=w622, "table"=w617, "connection reference"=w632) -> ("error out"=w624:errorcluster, "connection reference out"=w623:T9)  [unwired: 4 in]
              n64 = case shown="True" w633 {
                tunnel: w624 -> [w634 w654]
                tunnel: w623 -> [_ w653]
                tunnel: w622 -> [_ w644]
                tunnel: w621 -> [_ w650]
                tunnel: [w634 w648] -> w630
                tunnel: w617 -> [_ w646]
                tunnel: w616 -> [_ w642]
                frame False {
                  # "PLC com nok no updates"
                }
                frame True {
                  w635 = i16 1  # precision
                  # "Updating timer \nand pressure values\ncontinuesly"
                  # "Alarm Status"
                  # "PLC com OK alaram Update"
                  n65 = Boolean Array To Number(Boolean array=w650) -> (number=w651:u32)
                  n66 = Unbundle By Name(w642) -> ("MR Retn Tmr"=w641:dbl, "Holding Tmr"=w640:dbl, "1st Pressure"=w639:dbl, "2nd Pressure"=w638:dbl)
                  n67 = call <vilib>:"DB Tools Update Data.vi"("data"=w651, "error in (no error)"=w654, "columns"=w644, "table"="ALARM_STATUS", "connection reference"=w653) -> ("error out"=w649:errorcluster, "connection reference out"=w647:T9)  [unwired: 5 in]
                  n68 = Build Array(w641, w640, w639, w638) -> (w637:dbl[])
                  n69 = Number To Fractional String(number=w637, precision (6)=w635) -> (F-format string=w636:string[])  [unwired: 2 in]
                  n70 = for {
                    tunnel: w647 -> [w661]
                    tunnel: w646 -> [w660]
                    tunnel: "WHERE Sr_No = %s" ("condition") -> [w659]
                    tunnel: w649 -> [w663]
                    tunnel: [w662] -> w648
                    tunnel: w644 -> [w657]
                    tunnel: string[] ["2", "3", "4", "5"] -> [w656] mode=indexing
                    tunnel: w636 -> [w655] mode=indexing
                    n71 = Format Into String(format string=w659, w656) -> (resulting string=w658:string)  [unwired: 2 in, 1 out]
                    n72 = call <vilib>:"DB Tools Update Data.vi"("condition"=w658, "data"=w655, "error in (no error)"=w663, "columns"=w657, "table"=w660, "connection reference"=w661) -> ("error out"=w662:errorcluster)  [unwired: 4 in, 1 out]
                  }
                }
              }
            }
            n73 = call <vilib>:"Clear Errors.vi"("error in (no error)"=w610) -> ("error out"=w612:errorcluster)  [unwired: 5 in, 1 out]
          }
        }
        "Stop from Main" <- w517
        n74 = Wait (ms)(milliseconds to wait=u32 1000) -> ()  [unwired: 1 out]
      }
      n75 = while {
        tunnel: w67 -> [w292]
        tunnel: w68 -> [w295]
        tunnel: [w291] -> w69
        tunnel: w43 -> [w304]
        shift-right: [w303] -> _
        shift-left: w61 -> [w302]
        tunnel: w33 -> [w298]
        shift-right: [w301] -> _
        shift-left: Processing_enum."Inita" -> [w300]
        shift-right: [w293] -> _
        shift-left: w56 -> [w299]
        shift-right: [w297] -> _
        shift-left: FALSE -> [w296]
        tunnel: w56 -> [w290]
        stop <- w291 stop-if-true
        # "logging Data"
        n76 = case shown="\"Product_Rej_Count\"" w300 {
          tunnel: w292 -> [w307 w319 w358 w421]
          tunnel: w295 -> [_ w317 _ _]
          tunnel: [w307 w311 w350 w414] -> w291
          tunnel: w304 -> [_ _ w367 w427]
          tunnel: [w308 w314 w366 w426] -> w303
          tunnel: w302 -> [w308 w318 w366 w426]
          tunnel: [Processing_enum."PLC_stat" w321 w363 Processing_enum."PLC_stat"] -> w301
          tunnel: w299 -> [w309 w313 w354 w418]
          tunnel: [w309 w322 w353 w417] -> w293
          tunnel: w298 -> [_ _ w356 w422]
          tunnel: [w306 w320 FALSE FALSE] -> w297
          tunnel: w296 -> [w306 _ w362 _]
          tunnel: w290 -> [_ w310 _ _]
          frame "Inita", Default {
          }
          frame "PLC_stat" {
            # "PLC communication and Alarm"
            n77 = Dequeue Element(queue=w317, timeout in ms (-1)=50, error in (no error)=w319) -> (element=w323:T5[], timed out?=w315:bool, error out=w312:errorcluster)  [unwired: 1 out]
            n78 = case shown="False" w315 {
              tunnel: w323 -> [w327 _]
              tunnel: [w340 w348] -> w322
              tunnel: [w336 Processing_enum."PLC_stat"] -> w321
              tunnel: [w331 FALSE] -> w320
              tunnel: w319 -> [w329 _]
              tunnel: w318 -> [w328 w349]
              tunnel: [w327 w349] -> w314
              tunnel: w313 -> [_ w348]
              tunnel: [w325 w345] -> w311
              tunnel: w312 -> [w325 w345]
              tunnel: w310 -> [w324 _]
              frame False {
                (unwired) T3 {"Rejection code"=[FALSE, FALSE, FALSE, FALSE, FALSE, FALSE, FALSE, FALSE, FALSE, FALSE], "Production count"=[FALSE, FALSE, FALSE, FALSE, FALSE, FALSE, FALSE, FALSE, FALSE, FALSE], "Input"=[[FALSE, FALSE, FALSE, FALSE, FALSE], [FALSE, FALSE, FALSE, FALSE, FALSE], [FALSE, FALSE, FALSE, FALSE, FALSE], [FALSE, FALSE, FALSE, FALSE, FALSE], [FALSE, FALSE, FALSE, FALSE, FALSE], [FALSE, FALSE, FALSE, FALSE, FALSE], [FALSE, FALSE, FALSE, FALSE, FALSE], [FALSE, FALSE, FALSE, FALSE, FALSE], [FALSE, FALSE, FALSE, FALSE, FALSE], [FALSE, FALSE, FALSE, FALSE, FALSE]]}
                n79 = Not Equal?(x=w328, y=w327) -> (x != y?=w330:T1)
                "Change Element" <- w330
                n80 = for {
                  tunnel: w329 -> [_]
                  tunnel: w330 -> [w344] mode=indexing
                  tunnel: [w343] -> w338 mode=indexing
                  tunnel: [w342] -> w337 mode=indexing
                  tunnel: [w341] -> w326 mode=indexing
                  n81 = Unbundle By Name(w344) -> ("REJECTION COUNT"=w343:bool, "CYCLE COUNT"=w342:bool, "Input"=w341:bool[])
                }
                n82 = Build Array(w338, w337) -> (w339:bool[][])
                n83 = Or Array Elements(Boolean array=w339) -> (logical OR=w333:bool)
                n84 = Or Array Elements(Boolean array=w326) -> (logical OR=w331:bool)
                n85 = Or(x=w333, y=w331) -> (x .or. y?=w332:bool)
                n86 = Bundle By Name(cluster=w324, "Rejection code"=w338, "Production count"=w337, "Input"=w326) -> (w340:T3)
                n87 = Select(t=Processing_enum."Product_Rej_Count", s=w332, f=Processing_enum."PLC_stat") -> (s? t:f=w336:T4)
                "Deq Element" <- w327
              }
              frame True {
              }
            }
          }
          frame "Product_Rej_Count" {
            w352 = bool[] [FALSE, FALSE, FALSE, FALSE, FALSE, FALSE]  # Production count
            # "PLC PRODUCT/CYCLE COUNT AND REJECTION COUNT"
            n88 = Unbundle By Name(w354) -> ("Rejection code"=w365:bool[], "Production count"=w364:bool[])
            n89 = call "Shift_Logic.vi"("error in (no error)"=w358, "Time Stamp IN"=w356) -> ("error out"=w357:errorcluster, "Shift"=w355:i32)  [unwired: 8 in]
            "Shift" <- w355
            n90 = Bundle By Name(cluster=w354, "Production count"=w352, "Rejection code"=w352) -> (w353:T3)
            n91 = for {
              tunnel: w357 -> [w379]
              tunnel: [w374] -> w368
              tunnel: w366 -> [w377] mode=indexing
              tunnel: w367 -> [w378]
              tunnel: w365 -> [w376] mode=indexing
              tunnel: w364 -> [w370] mode=indexing
              tunnel: w355 -> [w369]
              n92 = case shown="True" w376 {
                tunnel: w379 -> [w397 w405]
                tunnel: [w397 w404] -> w375
                tunnel: w378 -> [w395 w403]
                tunnel: w377 -> [w396 w398]
                tunnel: [w396 w398] -> w373
                tunnel: [w395 w400] -> w372
                tunnel: w369 -> [w394 w399]
                tunnel: [w394 w399] -> w371
                frame False {
                }
                frame True {
                  # "Check Reject data in SQL"
                  # "Rejection count add"
                  n93 = Unbundle By Name(w398) -> ("REJECTION COUNT"=w402:u32)
                  n94 = Not Equal To 0?(x=w402) -> (x != 0?=w401:bool)
                  n95 = case shown="True" w401 {
                    tunnel: w405 -> [w407 w413]
                    tunnel: [w407 w412] -> w404
                    tunnel: w403 -> [w406 w411]
                    tunnel: w399 -> [_ w410]
                    tunnel: [w406 w409] -> w400
                    tunnel: w398 -> [_ w408]
                    frame False {
                    }
                    frame True {
                      n96 = call "Rejection_SQL_data_fetch.vi"("error constant"=w413, "Cycle Data"=w408, "Current Shift"=w410, "connection reference"=w411) -> ("error out 3"=w412:errorcluster, "Refnum out 2"=w409:T9)  [unwired: 3 in, 1 out]
                    }
                  }
                }
              }
              n97 = case shown="True" w370 {
                tunnel: w375 -> [w380 w387]
                tunnel: [w380 w386] -> w374
                tunnel: w372 -> [_ w385]
                tunnel: w373 -> [_ w381]
                tunnel: w371 -> [_ w382]
                frame False {
                }
                frame True {
                  # "Check Cycle count data in SQL"
                  # "Product count add"
                  n98 = Unbundle By Name(w381) -> ("CYCLE COUNT"=w384:u32)
                  n99 = Not Equal To 0?(x=w384) -> (x != 0?=w383:bool)
                  n100 = case shown="True" w383 {
                    tunnel: w387 -> [w388 w393]
                    tunnel: [w388 w392] -> w386
                    tunnel: w385 -> [_ w391]
                    tunnel: w382 -> [_ w390]
                    tunnel: w381 -> [_ w389]
                    frame False {
                    }
                    frame True {
                      n101 = call "Production_count_SQL_data_fetch.vi"("Current Shift"=w390, "error in (no error)"=w393, "Cycle Data"=w389, "Refnum in"=w391) -> ("error out"=w392:errorcluster)  [unwired: 5 in]
                    }
                  }
                }
              }
            }
            n102 = Merge Errors(w358, w368) -> (w351:errorcluster)
            n103 = call <vilib>:"Clear Errors.vi"("error in (no error)"=w351) -> ("error out"=w350:errorcluster)  [unwired: 5 in, 1 out]
            n104 = Select(t=Processing_enum."Break_down", s=w362, f=Processing_enum."PLC_stat") -> (s? t:f=w363:T4)
          }
          frame "Break_down" {
            w416 = bool[][] [[FALSE, FALSE, FALSE, FALSE, FALSE], [FALSE, FALSE, FALSE, FALSE, FALSE], [FALSE, FALSE, FALSE, FALSE, FALSE], [FALSE, FALSE, FALSE, FALSE, FALSE], [FALSE, FALSE, FALSE, FALSE, FALSE], [FALSE, FALSE, FALSE, FALSE, FALSE]]  # Input
            # "PLC Break_down"
            n105 = Unbundle By Name(w418) -> ("Input"=w423:bool[][])
            n106 = call "Shift_Logic.vi"("error in (no error)"=w421, "Time Stamp IN"=w422) -> ("error out"=w420:errorcluster, "Shift"=w419:i32)  [unwired: 8 in]
            n107 = for {
              tunnel: w420 -> [w435]
              tunnel: [w432] -> w428
              tunnel: w426 -> [w433] mode=indexing
              tunnel: w427 -> [w434]
              tunnel: w423 -> [w429] mode=indexing
              tunnel: w419 -> [w430]
              n108 = Or Array Elements(Boolean array=w429) -> (logical OR=w431:bool)
              n109 = case shown="True" w431 {
                tunnel: w435 -> [w438 w453]
                tunnel: [w438 w444] -> w432
                tunnel: w434 -> [w436 w452]
                tunnel: w433 -> [w437 w447]
                tunnel: [w437 w447] -> _
                tunnel: [w436 w451] -> _
                tunnel: w430 -> [_ w454]
                tunnel: w429 -> [_ w443]
                frame False {
                }
                frame True {
                  # "output for ack on PLC"
                  # "Check Reject data in SQL"
                  # "Break_down status update"
                  n110 = Unbundle By Name(w447) -> ("Input"=w457:bool[], "CID"=w456:string, "PRODUCT_CODE"=w458:i16)
                  "CID" <- w456
                  "Input" <- w457
                  n111 = Number To Decimal String(number=w458) -> (decimal integer string=w455:string)  [unwired: 1 in]
                  n112 = for {
                    tunnel: w457 -> [w469] mode=indexing
                    tunnel: w456 -> [w468]
                    tunnel: w455 -> [w467]
                    tunnel: w454 -> [w466]
                    tunnel: w453 -> [w464]
                    tunnel: [w463] -> w448
                    tunnel: w452 -> [w462]
                    tunnel: [w461] -> w451
                    tunnel: w443 -> [w460] mode=indexing
                    i -> [w465]
                    n113 = case shown="True" w460 {
                      tunnel: w469 -> [_ w481]
                      tunnel: w468 -> [_ w480]
                      tunnel: w467 -> [_ w479]
                      tunnel: w466 -> [_ w478]
                      tunnel: w465 -> [_ w477]
                      tunnel: w464 -> [w471 w475]
                      tunnel: [w471 w474] -> w463
                      tunnel: w462 -> [w470 w473]
                      tunnel: [w470 w472] -> w461
                      frame False {
                      }
                      frame True {
                        n114 = Increment(x=w477) -> (x+1=w476:i32)
                        n115 = case shown="False" w481 {
                          tunnel: w480 -> [w483 w497]
                          tunnel: w479 -> [_ _]
                          tunnel: w478 -> [_ w498]
                          tunnel: w476 -> [w482 w492]
                          tunnel: w475 -> [w487 w502]
                          tunnel: [w486 w501] -> w474
                          tunnel: w473 -> [w485 w500]
                          tunnel: [w484 w499] -> w472
                          frame False {
                            # "trigger Closed"
                            n116 = call "Demo_Andon get max ID with Breakdwn ID.vi"("error in (no error)"=w487, "Station No."=w483, "BREAKDOWN ID"=w482, "Refnum in"=w485) -> ("error out"=w491:errorcluster, "TABLE NAME"=w489:string, "Refnum out"=w490:T9, "CONDITION string"=w488:string)  [unwired: 2 in, 1 out]
                            n117 = call "Demo_CLOSE_SQL_DATA.vi"("error in (no error)"=w491, "TABLE NAME"=w489, "CONDITION string"=w488, "Refnum in"=w490) -> ("error out"=w486:errorcluster, "Refnum out"=w484:T9)  [unwired: 6 in]
                          }
                          frame True {
                            # "Breakdown ID"
                            # "Trigger"
                            n118 = call "Demo_Andon get max ID.vi"("error in (no error)"=w502, "Station No."=w497, "Refnum in"=w500) -> ("error out"=w496:errorcluster, "TABLE NAME"=w493:string, "ID MAX"=w494:i32, "Refnum out"=w495:T9)  [unwired: 5 in]
                            n119 = call "Demo_TRIGGER_SQL_DATA.vi"("STATION ID_CID"=w497, "TABLE NAME"=w493, "BREAKDOWN ID"=w492, "error in (no error)"=w496, "ID MAX"=w494, "Shift"=w498, "Refnum in"=w495) -> ("error out"=w501:errorcluster, "Refnum out"=w499:T9)  [unwired: 3 in]
                          }
                        }
                      }
                    }
                    n120 = Wait (ms)(milliseconds to wait=u32 20) -> ()  [unwired: 1 out]
                  }
                  n121 = Unbundle By Name(w447) -> ("ip address's"=w445:string, "Input"=w446:bool[])
                  n122 = call-poly <vilib>:"EthernetIP SLC500 Write.vi"("File Number"=u16 24, "Network Path"=w445, "Element Number"=u16 2, "Data"=w446, "error in"=w448) -> ("Session out"=w439:T13, "error out"=w441:errorcluster)  [unwired: 9 in]
                  n123 = call <vilib>:"EthernetIP Close Session.vi"("error in"=w441, "Session in"=w439) -> ("error out"=w440:errorcluster)  [unwired: 9 in]
                  n124 = call <vilib>:"Clear Errors.vi"("error in (no error)"=w440) -> ("error out"=w444:errorcluster)  [unwired: 5 in, 1 out]
                  n125 = Wait (ms)(milliseconds to wait=u32 20) -> ()  [unwired: 1 out]
                }
              }
            }
            n126 = Bundle By Name(cluster=w418, "Input"=w416) -> (w417:T3)
            n127 = Merge Errors(w421, w428) -> (w415:errorcluster)
            n128 = call <vilib>:"Clear Errors.vi"("error in (no error)"=w415) -> ("error out"=w414:errorcluster)  [unwired: 5 in, 1 out]
          }
        }
        "Cluster" <- w293
        n129 = Wait (ms)(milliseconds to wait=u32 100) -> ()  [unwired: 1 out]
        "STATE" <- w300
      }
      n130 = while {
        shift-right: [w131] -> w34
        shift-left: w41 -> [w132]
        shift-right: [w129] -> _
        shift-left: w55 -> [w130]
        shift-right: [w126] -> _
        shift-left: w38 -> [w128]
        tunnel: w33 -> [w121]
        stop <- w122 stop-if-true
        w124 = Oven_State."Stop"  # Enum
        # "1=no error, 1=log enable, values..."
        # "Oven PLC"
        n131 = case shown="\"Log data\"" w128 {
          tunnel: w132 -> [w139 w162 w212 w236 w280]
          tunnel: [w138 w156 w211 w231 w283] -> w131
          tunnel: w130 -> [w136 w159 w210 w234 w282]
          tunnel: [w135 w160 w210 w234 w282] -> w129
          tunnel: [w133 w153 w208 w240 w285] -> w123
          tunnel: [_ _ _ _ TRUE] -> w122
          tunnel: w121 -> [_ _ _ w238 _]
          frame "Initialise" {
            w133 = Oven_State."PLC read"  # Enum
            n132 = Unbundle By Name(w136) -> ("IP Address"=w137:string[])
            n133 = for {
              tunnel: w139 -> [w145]
              tunnel: [w142] -> w138
              tunnel: w137 -> [w144] mode=indexing
              tunnel: [w141] -> w134 mode=indexing
              n134 = call <vilib>:"Clear Errors.vi"("error in (no error)"=w145) -> ("error out"=w147:errorcluster)  [unwired: 5 in, 1 out]
              n135 = call-poly <vilib>:"Create Modbus Instance.vi"("error in"=w147, "connect timeout ms"=1000, "address"=w144) -> ("error out"=w143:errorcluster, "TCP master instance"=w140:refnum<class "Modbus Master.lvclass">)  [unwired: 7 in]
              n136 = case shown="Error" w143 {
                selector: w143 -> [w149 w151]
                tunnel: [w149 w150] -> w142
                tunnel: [w148 w152] -> w141
                tunnel: w140 -> [w148 _]
                frame No Error {
                }
                frame Error {
                  w152 = refnum<class "Modbus Master.lvclass"> refnum  # TCP master instance
                  n137 = call <vilib>:"Clear Errors.vi"("error in (no error)"=w151) -> ("error out"=w150:errorcluster)  [unwired: 5 in, 1 out]
                }
              }
            }
            n138 = Bundle By Name(cluster=w136, "PLC ref"=w134) -> (w135:T10)
          }
          frame "PLC read" {
            w153 = Oven_State."Live Update"  # Enum
            # "PLC Read Data case"
            n139 = Unbundle By Name(w159) -> ("IP Address"=w158:string[], "PLC ref"=w155:refnum<class "Modbus Master.lvclass">[])
            n140 = for {
              tunnel: w158 -> [w176] mode=indexing
              tunnel: [w175] -> w157 mode=indexing
              tunnel: w155 -> [w172] mode=indexing
              tunnel: [w168] -> w154 mode=indexing
              tunnel: w162 -> [w174]
              tunnel: [w177] -> w161
              w169 = u16 900  # starting address
              # "Need to add starting address"
              # "Oven PLC data read"
              n141 = call-dynamic "Read Holding Registers.vi"("error in"=w174, "number of inputs"=u16 36, "starting address"=w169, "Modbus master in"=w172) -> ("error out"=w173:errorcluster, "register values"=w165:u16[], "Modbus master out"=w171:refnum<class "Modbus Master.lvclass">)  [unwired: 5 in]
              n142 = Decimate 1D Array(w165) -> (w163:u16[])  [unwired: 1 out]
              n143 = Delete From Array(array=w163) -> (deleted portion=w167:u16, array with subset deleted=w166:u16[])  [unwired: 2 in]
              n144 = Build Array (concatenate)(w167, w166) -> (w164:u16[])
              n145 = case shown="Error" w173 {
                selector: w173 -> [w181 w193]
                tunnel: w171 -> [w182 w191]
                tunnel: [w182 w188] -> w175
                tunnel: [w181 w185] -> w177
                tunnel: w176 -> [_ w186]
                tunnel: w164 -> [w179 w183]
                tunnel: [w178 w184] -> w168
                frame No Error {
                  w180 = u16[] [1]  # array
                  n146 = Build Array (concatenate)(w180, w179) -> (w178:u16[])
                }
                frame Error {
                  n147 = call <vilib>:"Clear Errors.vi"("error in (no error)"=w193) -> ("error out"=w192:errorcluster)  [unwired: 5 in, 1 out]
                  n148 = call-dynamic "Shutdown.vi"("error in"=w192, "Modbus master in"=w191) -> ("error out"=w190:errorcluster)  [unwired: 9 in]
                  n149 = call <vilib>:"Clear Errors.vi"("error in (no error)"=w190) -> ("error out"=w189:errorcluster)  [unwired: 5 in, 1 out]
                  n150 = call-poly <vilib>:"Create Modbus Instance.vi"("error in"=w189, "connect timeout ms"=1000, "address"=w186) -> ("error out"=w185:errorcluster, "TCP master instance"=w188:refnum<class "Modbus Master.lvclass">)  [unwired: 7 in]
                  n151 = case shown="Error" w185 {
                    tunnel: [w195 u16[] [0, 0, 0, 0, 0, 0, 0, 0, 0, 0, 0, 0, 0, 0, 0, 0, 0, 0, 0] ("register values")] -> w184
                    tunnel: w183 -> [w196 _]
                    frame No Error {
                      w194 = u16[] [1]  # array
                      n152 = Build Array (concatenate)(w194, w196) -> (w195:u16[])
                    }
                    frame Error {
                    }
                  }
                }
              }
            }
            "Oven Values" <- w154
            n153 = Bundle By Name(cluster=w159, "Oven Data"=w154, "PLC ref"=w157) -> (w160:T10)
            n154 = call <vilib>:"Clear Errors.vi"("error in (no error)"=w161) -> ("error out"=w156:errorcluster)  [unwired: 5 in, 1 out]
          }
          frame "Live Update" {
            w199 = 1  # index (row)
            w203 = string[] ["1", "Top_zone_1", "Top_zone_2", "Top_zone_3", "Top_zone_4", "Top_zone_5", "Top_zone_6", "Top_zone_7", "Top_zone_8", "Bottom_zone_1", "Bottom_zone_2", "Bottom_zone_3", "Bottom_zone_4", "Bottom_zone_5", "Bottom_zone_6", "Bottom_zone_7", "Bottom_zone_8", "Heating_time"]  # Array
            w205 = Oven_State."PLC read"  # Enum
            w206 = Oven_State."Log data"  # Enum
            # "Remove = 1=log enable"
            # "chn age to log"
            # "Change row names"
            # "Live Oven data"
            n155 = Unbundle By Name(w210) -> ("Oven Number Txx"=w207:string[], "SQL connection"=w204:T9, "Oven Data"=w202:u16[][])
            n156 = Transpose 2D Array(2D array=w202) -> (transposed array=w201:u16[][])
            n157 = Delete From Array(array=w201, index (row)=w199) -> (array with subset deleted=w200:u16[][])  [unwired: 2 in, 1 out]
            n158 = for {
              shift-right: [w215] -> w211
              shift-left: w212 -> [w221]
              tunnel: w207 -> [w213]
              tunnel: w204 -> [w219]
              tunnel: w200 -> [w214] mode=indexing
              tunnel: w203 -> [w218] mode=indexing
              n159 = Format Into String(format string="WHERE Sr_No = '%s'" ("condition"), w218) -> (resulting string=w217:string)  [unwired: 2 in, 1 out]
              n160 = for {
                tunnel: w219 -> [w227]
                tunnel: w217 -> [w225]
                tunnel: w214 -> [w224] mode=indexing
                tunnel: w213 -> [w223] mode=indexing
                tunnel: w221 -> [w229]
                tunnel: [w228] -> w220
                n161 = Build Array(w223) -> (w222:string[])
                n162 = call <vilib>:"DB Tools Update Data.vi"("condition"=w225, "data"=w224, "error in (no error)"=w229, "columns"=w222, "table"="dbo.OVEN_CON_STATUS", "connection reference"=w227) -> ("error out"=w228:errorcluster)  [unwired: 4 in, 1 out]
                "Oven live Sql Error" <- w228
              }
              n163 = call <vilib>:"Clear Errors.vi"("error in (no error)"=w220) -> ("error out"=w215:errorcluster)  [unwired: 5 in, 1 out]
            }
            n164 = call "Elapsed Time"() -> ("Elapsed Time (s)"=→"LOG Elapsed Time":dbl, "Time has Elapsed"=w209:bool)  [unwired: 12 in, 6 out]
            n165 = Select(t=w206, s=w209, f=w205) -> (s? t:f=w208:T8)
          }
          frame "Log data" {
            w240 = Oven_State."PLC read"  # Enum
            # "SQL Data log"
            n166 = call "Shift_Logic.vi"("error in (no error)"=w236, "Time Stamp IN"=w238) -> ("error out"=w235:errorcluster, "Shift"=w237:i32)  [unwired: 8 in]
            n167 = Unbundle By Name(w234) -> ("SQL connection"=w239:T9, "Oven Data"=w233:u16[][], "Oven Number"=w232:string[], "Oven NAME"=w230:string[])
            n168 = for {
              tunnel: w233 -> [w250] mode=indexing
              tunnel: w235 -> [w254]
              tunnel: [w253] -> w241
              tunnel: w239 -> [w251]
              tunnel: w237 -> [w249]
              tunnel: w234 -> [w248]
              tunnel: w232 -> [w247] mode=indexing
              tunnel: w230 -> [w244]
              i -> [w243]
              # "Save data in SQL"
              n169 = Delete From Array(array=w250, index=0) -> (deleted portion=w252:u16, array with subset deleted=w245:u16[])  [unwired: 1 in]
              n170 = Index Array(array=w244, index=w243) -> (element=w242:string)
              n171 = case shown="1" w252 {
                tunnel: w254 -> [w255 w266]
                tunnel: [w255 w263] -> w253
                tunnel: w251 -> [_ w265]
                tunnel: w249 -> [_ w261]
                tunnel: w248 -> [_ _]
                tunnel: w247 -> [_ w260]
                tunnel: w245 -> [_ w259]
                tunnel: w242 -> [_ w256]
                frame 0, Default {
                  # "PLC IS IN ERROR--- SO NO LOG FOR IT"
                }
                frame 1 {
                  # "plc IS IN NO ERROR"
                  n172 = Delete From Array(array=w259, index=0) -> (deleted portion=w257:u16, array with subset deleted=w258:u16[])  [unwired: 1 in]
                  n173 = Merge Errors(w266) -> (w264:errorcluster)
                  n174 = case shown="1" w257 {
                    tunnel: w265 -> [_ w271]
                    tunnel: w264 -> [w267 w277]
                    tunnel: [w267 w276] -> w263
                    tunnel: w261 -> [_ w274]
                    tunnel: w260 -> [_ w272]
                    tunnel: w258 -> [_ w269]
                    tunnel: w256 -> [_ w268]
                    frame 0, Default {
                      # "loGING IS DISABLED"
                    }
                    frame 1 {
                      w270 = string[] ["STATION_ID", "DATE", "SHIFT", "PLAN_DATE", "PRODUCT_CODE", "Top_zone_1", "Top_zone_2", "Top_zone_3", "Top_zone_4", "Top_zone_5", "Top_zone_6", "Top_zone_7", "Top_zone_8", "Bottom_zone_1", "Bottom_zone_2", "Bottom_zone_3", "Bottom_zone_4", "Bottom_zone_5", "Bottom_zone_6", "Bottom_zone_7", "Bottom_zone_8", "Heating_time", "MR_RETURN_TIME", "HOLDING_TIME", "PRESSURE_1st", "PRESSURE_2nd", "STATION_NAME"]  # Oven para
                      # "Change table name"
                      # "SQL oven data in 10 minute LOG"
                      n175 = local read "PLC Data"() -> (w273:T5[])
                      n176 = call "Oven_Logs.vi"("Oven Staion NAME"=w268, "SQl IN"=w271, "Oven Data"=w269, "Oven Staion ID"=w272, "Shift"=w274, "PLC Data"=w273) -> ("output cluster"=w275:T2)  [unwired: 5 in]
                      "output cluster" <- w275
                      n177 = call <vilib>:"DB Tools Insert Data.vi"("data"=w275, "error in (no error)"=w277, "columns"=w270, "table"="OVEN_LOG", "connection reference"=w271) -> ("error out"=w276:errorcluster)  [unwired: 5 in, 1 out]
                    }
                  }
                }
              }
              "Oven LOG SQL Error" <- w253
            }
            n178 = call <vilib>:"Clear Errors.vi"("error in (no error)"=w241) -> ("error out"=w231:errorcluster)  [unwired: 5 in, 1 out]
          }
          frame "Stop" {
            w285 = Oven_State."Stop"  # Enum
            # "STOP LOOP"
            n179 = Unbundle By Name(w282) -> ("PLC ref"=w281:refnum<class "Modbus Master.lvclass">[])
            n180 = call <vilib>:"Clear Errors.vi"("error in (no error)"=w280) -> ("error out"=w279:errorcluster)  [unwired: 5 in, 1 out]
            n181 = for {
              shift-right: [w289] -> w283
              shift-left: w279 -> [w288]
              tunnel: w281 -> [w286] mode=indexing
              n182 = call-dynamic "Shutdown.vi"("error in"=w288, "Modbus master in"=w286) -> ("error out"=w287:errorcluster)  [unwired: 9 in]
              n183 = call <vilib>:"Clear Errors.vi"("error in (no error)"=w287) -> ("error out"=w289:errorcluster)  [unwired: 5 in, 1 out]
            }
          }
        }
        n184 = local read "Stop from Main"() -> (w125:bool)
        n185 = Wait (ms)(milliseconds to wait=u32 5000) -> ()  [unwired: 1 out]
        n186 = Select(t=w124, s=w125, f=w123) -> (s? t:f=w126:T8)
      }
      n187 = call <vilib>:"Clear Errors.vi"("error in (no error)"=w110) -> ("error out"=w109:errorcluster)  [unwired: 5 in, 1 out]
      n188 = Flush Queue(queue=w113, error in (no error)=w109) -> (queue out=w114:refnum<queue>, error out=w115:errorcluster)  [unwired: 1 out]
      n189 = Release Queue(queue=w114, error in (no error)=w115) -> (error out=w108:errorcluster)  [unwired: 1 in, 2 out]
      n190 = Merge Errors(w34, w108, w69) -> (w60:errorcluster)
      n191 = call <vilib>:"Clear Errors.vi"("error in (no error)"=w60) -> ("error out"=w59:errorcluster)  [unwired: 5 in, 1 out]
      n192 = call "Stall Data Flow.vim"("value in"=w59, "milliseconds to wait"=u32 1000) -> ("value out"=w58:errorcluster)  [unwired: 1 out]
      n193 = call <vilib>:"DB Tools Close Connection.vi"("error in (no error)"=w58, "connection reference"=w64) -> ("error out"=w65:errorcluster)  [unwired: 5 in]
    }
  }
  n194 = call <vilib>:"Clear Errors.vi"("error in (no error)"=w4) -> ("error out"=w5:errorcluster)  [unwired: 5 in, 1 out]
  n195 = property class="App"(error in=w5) -> (error out=w14:errorcluster, "App.Kind"=w13:T6)  [unwired: 1 in, 1 out]
  n196 = case shown="\"Run Time System\"" w13 {
    tunnel: [w664 w667] -> _
    tunnel: w14 -> [w665 w667]
    frame "Run Time System" {
      n197 = control-ref of="This VI"() -> (w666:refnum<vi>)
      n198 = invoke class="VI" method="FP.Close"(reference=w666, error in=w665) -> (error out=w664:errorcluster)  [unwired: 1 in, 2 out]
    }
    frame "Development System", Default {
    }
  }
